vi "Begin.vi"(8 "error in":errorcluster) -> (0 "error out":errorcluster)   [LabVIEW 2017]
doc: "Called before other user functions, this VI is expected to open initial I/O refnums, load in file data, and do all program initialization. Notice that the <B>error out</B> terminal is simply used for data flow. Wiring it to other structures or subVIs ensures that this VI runs first."
uses:
  <vilib>/Rock Robotics/WPI/DriverStation/WPI_DriverStationRobotMode2.ctl
  <vilib>/Rock Robotics/WPI/Joystick/WPI_JoystickDeviceEnum.ctl
  Drive/Drive Notifier.ctl
  Drive/Drive Control Type.ctl
  Lift/Lift Notifier.ctl
  Lift/Lift Control Type.ctl
  Lift/Lift Enum States.ctl
  RPED/RPED Notifier.ctl
  RPED/RPED Control Type.ctl
  LEDs/LED Notifier.ctl
  LEDs/LED Control Type.ctl
  <vilib>/Rock Robotics/WPI/Solenoid/WPI_SolenoidChannel.ctl
  Intake Rotation/Intake Rotation Notifier.ctl
  Intake Rotation/Intake Rotation Control Type.ctl
  Intake Rotation/Arm Enum States.ctl
  Intake/Intake Notifier.ctl
  Intake/Intake Control Type.ctl
  <vilib>/Rock Robotics/SystemInterfaces/DIO/FPGA_DIOChannel.ctl
  <vilib>/Rock Robotics/WPI/ThirdParty/Phoenix-LabVIEW/Motor Controller/Controls/CTRE_Phoenix_MotorControl_FeedbackDevice.ctl
  <vilib>/Rock Robotics/SystemInterfaces/DIO/FPGA_DIOPWMChannel.ctl
  <vilib>/Rock Robotics/WPI/ThirdParty/Phoenix-LabVIEW/Motor Controller/Controls/CTRE_Phoenix_MotorControl_ControlMode.ctl
  Robot Global Data.vi
  <vilib>/Rock Robotics/WPI/Solenoid/WPI_SolenoidOpenDouble.vi
  <vilib>/Rock Robotics/WPI/ThirdParty/Phoenix-LabVIEW/Pigeon IMU/CTRE_PigeonIMU_Open_CAN.vi
  <vilib>/Rock Robotics/WPI/Switch/WPI_SwitchOpenLimit.vi
  <vilib>/Rock Robotics/WPI/MotorControl/WPI_MotorControlOpen VictorSP.vi
  Utility VIs/Refnum Names.vi
  Drive/Drive Globals.vi
  Intake/Intake Globals.vi
  Lift/Lift Globals.vi
  RPED/RPED Globals.vi
  Intake Rotation/Intake Rotation Globals.vi
  LEDs/LED Globals.vi
  <vilib>/Rock Robotics/WPI/Utilities/WPI_GetSetVariantRefNum.vi
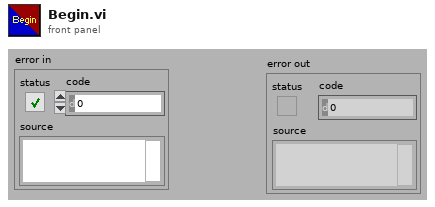
[diagram p1: front panel]
types:
  T1 = typedef "WPI_SolenoidChannel.ctl" = enum8{"Solenoid 0", "Solenoid 1", "Solenoid 2", "Solenoid 3", "Solenoid 4", "Solenoid 5", "Solenoid 6", "Solenoid 7", "Invalid"}
  T2 = enum16{"open", "replace", "create", "open or create", "replace or create", "replace or create with confirmation"}
  T3 = typedef "FPGA_DIOPWMChannel.ctl" = enum8{"PWM 0", "PWM 1", "PWM 2", "PWM 3", "PWM 4", "PWM 5", "PWM 6", "PWM 7", "PWM 8", "PWM 9", "PWM MXP 0", "PWM MXP 1", "PWM MXP 2", "PWM MXP 3", "PWM MXP 4", "PWM MXP 5", "PWM MXP 6", "PWM MXP 7", "PWM MXP 8", "PWM MXP 9", "Invalid"}
  T4 = typedef "FPGA_DIOChannel.ctl" = enum8{"DIO 0", "DIO 1", "DIO 2", "DIO 3", "DIO 4", "DIO 5", "DIO 6", "DIO 7", "DIO 8", "DIO 9", "DIO MXP 0", "DIO MXP 1", "DIO MXP 2", "DIO MXP 3", "DIO MXP 4", "DIO MXP 5", "DIO MXP 6", "DIO MXP 7", "DIO MXP 8", "DIO MXP 9", "DIO MXP 10", "DIO MXP 11", "DIO MXP 12", "DIO MXP 13", "DIO MXP 14", "DIO MXP 15", "SPI Port CS1", "SPI Port CS2", "SPI Port CS3", "SPI Port MISO", "SPI Port MOSI", "Invalid"}
  T5 = typedef "Intake Notifier.ctl" = cluster{"Intake Control Type":T6, "Step":i32, "In":bool, "Speed":dbl, "Out":bool, "Parameter 1":dbl, "Parameter 2":dbl, "Intake Notifier":refnum<notifier>, "Actuate Cube":bool, "Speed In":dbl, "Speed Out":dbl, "Load":bool, "Override":bool, "Exchange":bool, "Intake Open":bool}
  T6 = typedef "Intake Control Type.ctl" = enum16{"No Op", "In", "Out", "Test Mode", "Cube_In", "Cube_Out", "State_Change"}
  T7 = typedef "Intake Rotation Notifier.ctl" = cluster{"Step":i32, "Intake Rotation Control Type":T8, "Parameter 1":dbl, "Parameter 2":dbl, "Intake Rotation Notifier":refnum<notifier>, "Manual Up":bool, "Manual Down":bool, "Climb":bool, "Switch":bool, "Scale Low":bool, "Scale High":bool, "Stow":bool, "Load":bool, "Scale Mid":bool, "Exchange":bool, "Set Position":T9, "Portal":bool}
  T8 = typedef "Intake Rotation Control Type.ctl" = enum16{"No Op", "Manual Up", "Position", "Manual Down", "PositionAuto"}
  T9 = typedef "Arm Enum States.ctl" = enum16{"Current Position", "Climb", "Load", "Portal", "Switch", "Scale High", "Scale Mid", "Scale Low", "Exchange", "Stow"}
  T10 = typedef "LED Notifier.ctl" = cluster{"LED Control Type":T11, "Climbing":bool, "Auto Tracking":bool, "Ready for Cube Floor":bool, "Ready for Cube Portal":bool}
  T11 = typedef "LED Control Type.ctl" = enum16{"Off", "Waiting On Field", "Connected ", "Cube In Intake", "Climbing", "Auto Cube Capture", "Ready for Cube Floor", "Ready for Cube Portal"}
  T12 = typedef "RPED Notifier.ctl" = cluster{"RPED Control Type":T13, "Step":i32, "Left Forward":bool, "Right Forward":bool, "Parameter 1":dbl, "Parameter 2":dbl, "Parameter 3":dbl, "RPED Notifier":refnum<notifier>, "Left Back":bool, "Right Back":bool, "Right":bool, "Left":bool}
  T13 = typedef "RPED Control Type.ctl" = enum16{"No Op", "Left Manual", "Right Manual", "Time", "Left", "Right", "Left_Slow", "Right_Slow", "Left_Distance", "Right_Distance"}
  T14 = typedef "Lift Notifier.ctl" = cluster{"Lift Control Type":T15, "Step":i32, "Set Position":T16, "Climb":bool, "Switch":bool, "Scale Low":bool, "Scale Mid":bool, "Scale High":bool, "Stow":bool, "Load":bool, "Climb Actuation":bool, "Manual Up":bool, "Manual Down":bool, "Parameter 1":dbl, "Parameter 2":dbl, "Parameter 3":dbl, "Lift Notifier":refnum<notifier>, "Exchange":bool, "Brake":bool, "Portal":bool}
  T15 = typedef "Lift Control Type.ctl" = enum16{"No Op", "Position", "Climb Actuation", "Manual Up", "Manual Down", "PositionAuto", "Position_kP", "Position_Delay"}
  T16 = typedef "Lift Enum States.ctl" = enum16{"Climb", "Load", "Portal", "Switch", "Scale High", "Scale Mid", "Scale Low", "Exchange", "Stow", "Current Position"}
  T17 = typedef "Drive Notifier.ctl" = cluster{"Drive Control Type":T18, "Throttle":dbl, "Twist":dbl, "Step":i32, "High Gear":bool, "Parameter 1":dbl, "Parameter 2":dbl, "Parameter 3":dbl, "Drive Notifier":refnum<notifier>, "AutoTrack":bool}
  T18 = typedef "Drive Control Type.ctl" = enum16{"No_Op", "Basic Drive", "Time", "Heading", "Hybrid_Turn", "RC_Speed", "Switch_Slots", "AutoTrack_Cube", "Speed Test", "Turn_Cube", "To_Cube", "Wait", "Distance_Slow", "Distance", "D_H_Delay", "Distance_Delay", "Heading_Cap", "Heading_Tight", "Cube_Heading", "Distance_Ramp"}
  T19 = typedef "WPI_JoystickDeviceEnum.ctl" = enum16{"USB 0", "USB 1", "USB 2", "USB 3", "USB 4", "USB 5"}
  T20 = typedef "WPI_DriverStationRobotMode2.ctl" = enum16{"Autonomous Disabled", "Autonomous Enabled", "Teleop Disabled", "Teleop Enabled", "Disconnected", "Finish", "Test Disabled", "Test Enabled", "Emergency Stopped"}
  T21 = typedef "CTRE_Phoenix_MotorControl_FeedbackDevice.ctl" = i8
  T22 = typedef "CTRE_Phoenix_MotorControl_ControlMode.ctl" = u16
  T23 = typedef "WPI_MotorControlDeviceRef.ctl" = cluster{"DeviceStatus":errorcluster, "Type":T24, "PWM":cluster{"PWM Channel":T3, "DeadBand":T25}, "CAN":cluster{"Device Number":u8, "SetOutput VI Ref":variant, "GetOutput VI Ref":variant, "Enable VI Ref":variant, "Disable VI Ref":variant, "Data":variant}, "Invert":bool, "DIO PWM":cluster{"PWM \"Enable\" Channel":T3, "DIOChannel":T4, "PWM Rate":dbl}}
  T24 = typedef "WPI_MotorControlType.ctl" = enum16{"PWM", "CAN", "DIO PWM"}
  T25 = typedef "WPI_PWMDeadband.ctl" = cluster{"Name":string, "maxPositivePwm":i32, "minPositivePwm":i32, "centerPwm":i32, "maxNegativePwm":i32, "minNegativePwm":i32, "angularRange":u16}
  T26 = typedef "CTRE_PigeonIMU_DeviceRef.ctl" = cluster{"DeviceStatus":errorcluster, "Device Number":u8, "Type":T27, "Device ID":u32, "Handle":u64, "UsageFrame":u32, "Library Path":path}
  T27 = typedef "CTRE_PigeonIMU_ConnectionType.ctl" = u32
  T28 = typedef "CTRE_CANifier_DeviceRef.ctl" = cluster{"DeviceStatus":errorcluster, "Device Number":u8, "Handle":u64, "UsageFrame":u32, "Library Path":path}
  T29 = typedef "WPI_SwitchDevRef.ctl" = cluster{"DevStatus":errorcluster, "DIO Channel":T4, "CntIndex":T30, "Normally Closed":bool}
  T30 = typedef "FPGA_CounterCtrSystemIndex.ctl" = enum8{"Ctr 0", "Ctr 1", "Ctr 2", "Ctr 3", "Ctr 4", "Ctr 5", "Ctr 6", "Ctr 7", "Invalid"}
  T31 = typedef "WPI_SolenoidDevRef.ctl" = cluster{"DevStatus":errorcluster, "Pneumatics Control Module":u8, "Forward Solenoid Channel":T1, "Reverse Solenoid Channel":T1}
  T32 = typedef "WPI_DigitalInputDevRef.ctl" = cluster{"DevStatus":errorcluster, "DIO Channel":T4}
  T33 = typedef "WPI_CompressorDevRef.ctl" = cluster{"DevStatus":errorcluster, "Pneumatics Control Module":u8}
  T34 = typedef "WPI_JoystickDevRef.ctl" = cluster{"Device":T19}
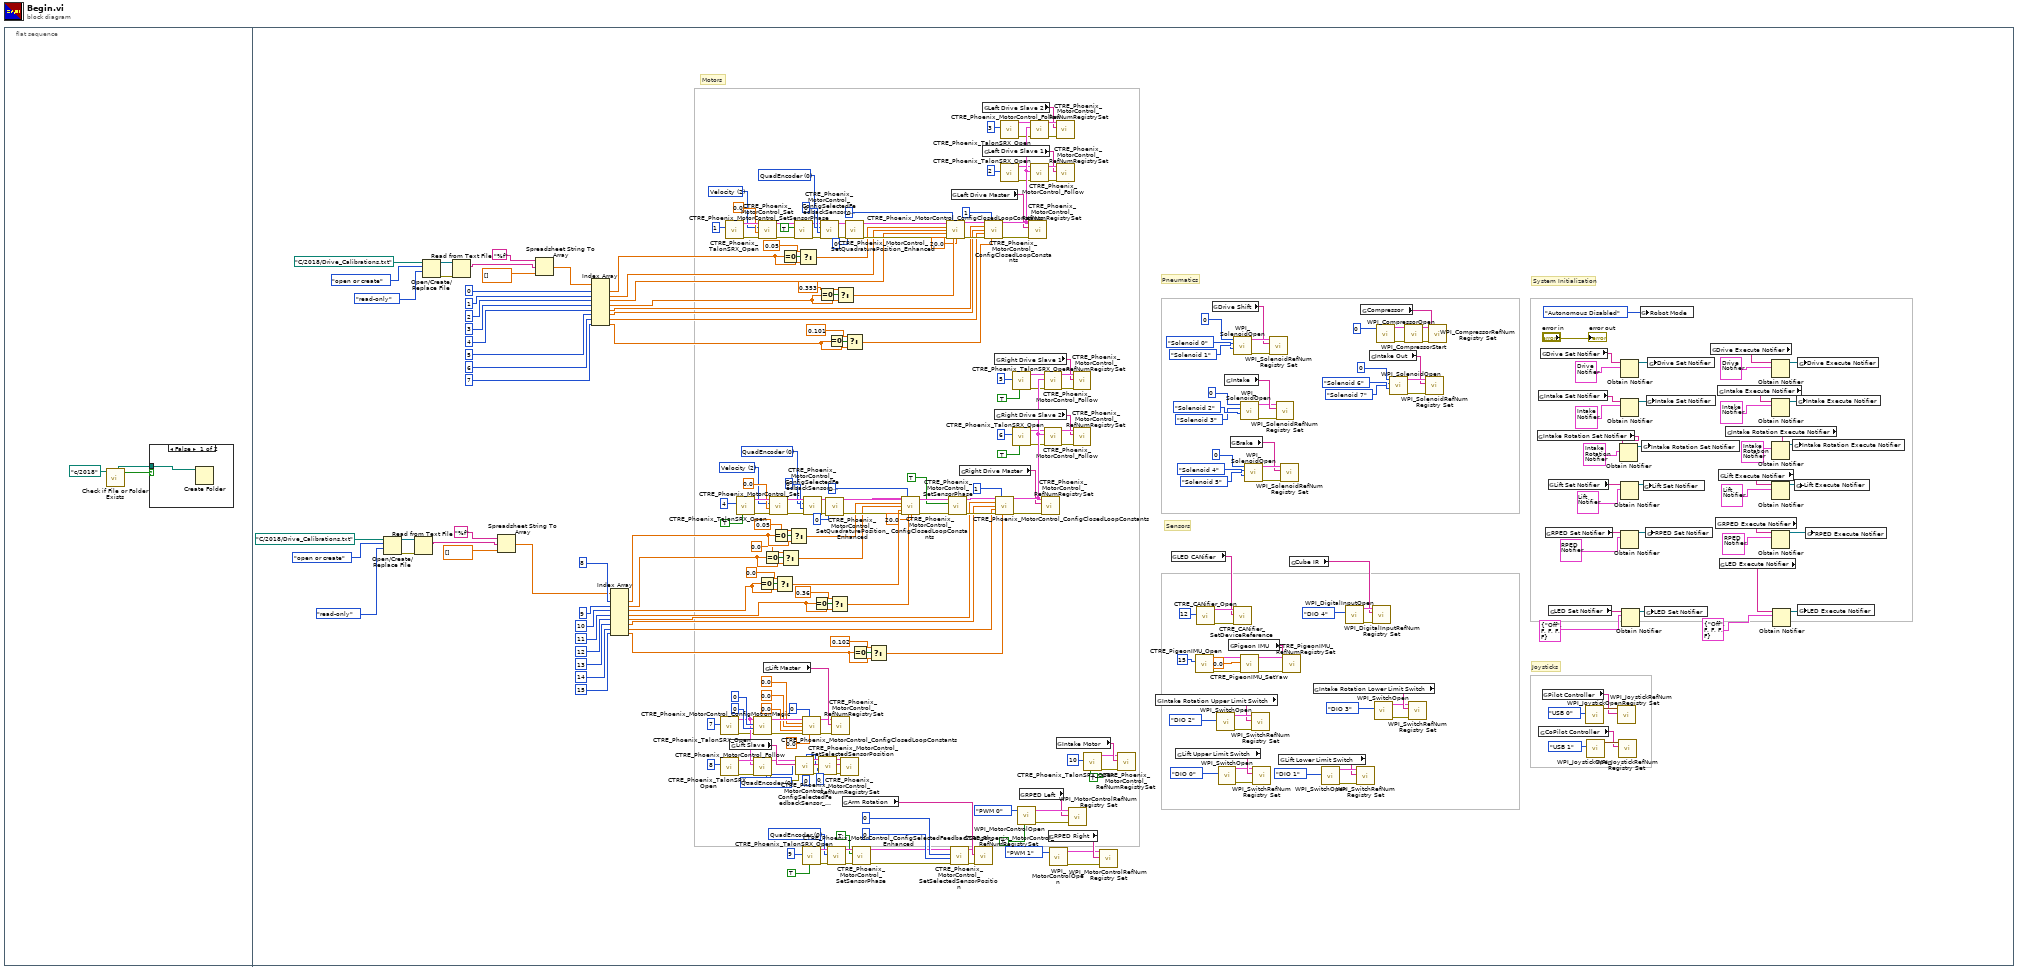
[diagram p0: block diagram]
diagram:
  n1 = flat-sequence {
    frame #0 {
      n2 = call <vilib>:"Check if File or Folder Exists.vi"("path"=path "c:/2018") -> ("file or folder exists?"=w3:bool, "dup path"=w1:path)  [unwired: 8 in, 1 out]
      n3 = case shown="False" w3 {
        tunnel: w1 -> [w4 _]
        frame False {
          n4 = Create Folder(path (use dialog)=w4) -> ()  [unwired: 2 in, 3 out]
        }
        frame True {
        }
      }
    }
    frame #1 {
      w111 = T21 0 items=["None"=-1, "QuadEncoder"=0, "Analog"=2, "Tachometer"=4, "Pulse Width Encoded Position"=8, "Sensor Sum (S0 + S1)"=9, "Sensor Difference (D0 - D1)"=10, "Remote Source 0"=11, "Remote Source 1"=12, "Software Emulated"=15] ("Feedback Device")
      w107 = T22 2 items=["PercentOutput"=0, "Position"=1, "Velocity"=2, "Current"=3, "Follower"=5, "MotionProfile"=6, "MotionMagic"=7, "MotionMagicArc"=8, "MotionProfileArc"=10, "Disabled"=15] ("Control Mode")
      w144 = T21 0 items=["None"=-1, "QuadEncoder"=0, "Analog"=2, "Tachometer"=4, "Pulse Width Encoded Position"=8, "Sensor Sum (S0 + S1)"=9, "Sensor Difference (D0 - D1)"=10, "Remote Source 0"=11, "Remote Source 1"=12, "Software Emulated"=15] ("Feedback Device")
      w140 = T22 2 items=["PercentOutput"=0, "Position"=1, "Velocity"=2, "Current"=3, "Follower"=5, "MotionProfile"=6, "MotionMagic"=7, "MotionMagicArc"=8, "MotionProfileArc"=10, "Disabled"=15] ("Control Mode")
      w204 = T21 0 items=["None"=-1, "QuadEncoder"=0, "Analog"=2, "Tachometer"=4, "Pulse Width Encoded Position"=8, "Sensor Sum (S0 + S1)"=9, "Sensor Difference (D0 - D1)"=10, "Remote Source 0"=11, "Remote Source 1"=12, "Software Emulated"=15] ("Feedback Device")
      w229 = T21 0 items=["None"=-1, "QuadEncoder"=0, "Analog"=2, "Tachometer"=4, "Pulse Width Encoded Position"=8, "Sensor Sum (S0 + S1)"=9, "Sensor Difference (D0 - D1)"=10, "Remote Source 0"=11, "Remote Source 1"=12, "Software Emulated"=15] ("Feedback Device")
      # "Joysticks"
      # "Sensors"
      # "System Initialization"
      # "Pneumatics"
      # "Motors"
      n5 = Open/Create/Replace File(file path (use dialog)=path "C:/2018/Drive_Calibrations.txt" ("file (use dialog)"), operation (0:open)=T2."open or create", access (0:read/write)=enum16{"read/write", "read-only", "write-only"}."read-only") -> (refnum out=w68:refnum<file>, error out=w67:errorcluster)  [unwired: 3 in, 1 out]
      n6 = Read from Text File(file (use dialog)=w68, error in=w67) -> (text=w61:string)  [unwired: 2 in, 3 out]
      n7 = Open/Create/Replace File(file path (use dialog)=path "C:/2018/Drive_Calibrations.txt" ("file (use dialog)"), operation (0:open)=T2."open or create", access (0:read/write)=enum16{"read/write", "read-only", "write-only"}."read-only") -> (refnum out=w59:refnum<file>, error out=w58:errorcluster)  [unwired: 3 in, 1 out]
      n8 = Read from Text File(file (use dialog)=w59, error in=w58) -> (text=w52:string)  [unwired: 2 in, 3 out]
      n9 = Spreadsheet String To Array(format string="%f", spreadsheet string=w61, array type (2D Dbl)=dbl[] []) -> (array=w60:dbl[])  [unwired: 1 in]
      n10 = Spreadsheet String To Array(format string="%f", spreadsheet string=w52, array type (2D Dbl)=dbl[] []) -> (array=w51:dbl[])  [unwired: 1 in]
      n11 = Index Array(array=w51, index #1=0 ("index"), index #2=1 ("index"), index #3=2 ("index"), index #4=3 ("index"), index #5=4 ("index"), index #6=5 ("index"), index #7=6 ("index"), index #8=7 ("index")) -> (element #1=w28:dbl, element #2=w84:dbl, element #3=w80:dbl, element #4=w23:dbl, element #5=w83:dbl, element #6=w82:dbl, element #7=w81:dbl, element #8=w19:dbl)
      n12 = Index Array(array=w60, index #1=8 ("index"), index #2=9 ("index"), index #3=10 ("index"), index #4=11 ("index"), index #5=12 ("index"), index #6=13 ("index"), index #7=14 ("index"), index #8=15 ("index")) -> (element #1=w49:dbl, element #2=w44:dbl, element #3=w41:dbl, element #4=w36:dbl, element #5=w71:dbl, element #6=w70:dbl, element #7=w69:dbl, element #8=w31:dbl)
      n13 = call <vilib>:"CTRE_Phoenix_TalonSRX_Open.vi"("Device Number"=u8 7) -> ("error out"=w263:errorcluster, "CAN Talon SRX Ref"=w264:T23)  [unwired: 9 in]
      n14 = call <vilib>:"CTRE_Phoenix_TalonSRX_Open.vi"("Device Number"=u8 8) -> ("error out"=w277:errorcluster, "CAN Talon SRX Ref"=w276:T23)  [unwired: 9 in]
      n15 = call <vilib>:"CTRE_Phoenix_TalonSRX_Open.vi"("Device Number"=u8 1) -> ("error out"=w117:errorcluster, "CAN Talon SRX Ref"=w118:T23)  [unwired: 9 in]
      n16 = global read "Refnum Names.vi" "Lift Slave"() -> (w279:string)
      n17 = call <vilib>:"CTRE_Phoenix_TalonSRX_Open.vi"("Invert"=TRUE, "Device Number"=u8 4) -> ("error out"=w155:errorcluster, "CAN Talon SRX Ref"=w156:T23)  [unwired: 8 in]
      n18 = call <vilib>:"CTRE_Phoenix_MotorControl_ConfigMotionMagic.vi"("error in (no error)"=w263, "Acceleration"=0, "Cruise Velocity"=0, "PhoenixMotorControlDevRef"=w264) -> ("error out"=w267:errorcluster, "PhoenixMotorControlDevRef"=w272:T23)  [unwired: 6 in]
      n19 = call <vilib>:"CTRE_Phoenix_MotorControl_Follow.vi"("error in (no error)"=w277, "Master Controller to Follow"=w264, "PhoenixMotorControlDevRef"=w276) -> ("error out"=w205:errorcluster, "PhoenixMotorControlDevRef"=w206:T23)  [unwired: 7 in]
      n20 = Equal To 0?(x=w41) -> (x = 0?=w42:bool)
      n21 = call <vilib>:"CTRE_Phoenix_MotorControl_Set.vi"("error in (no error)"=w117, "Output"=0.0, "Control Mode"=w107, "PhoenixMotorControlDevRef"=w118) -> ("error out"=w96:errorcluster, "PhoenixMotorControlDevRef"=w97:T23)  [unwired: 6 in]
      n22 = Equal To 0?(x=w44) -> (x = 0?=w45:bool)
      n23 = global read "Refnum Names.vi" "Lift Master"() -> (w280:string)
      n24 = call <vilib>:"CTRE_Phoenix_MotorControl_Set.vi"("error in (no error)"=w155, "Output"=0.0, "Control Mode"=w140, "PhoenixMotorControlDevRef"=w156) -> ("error out"=w151:errorcluster, "PhoenixMotorControlDevRef"=w152:T23)  [unwired: 6 in]
      n25 = Equal To 0?(x=w49) -> (x = 0?=w50:bool)
      n26 = Select(t=0.0, s=w42, f=w41) -> (s? t:f=w39:dbl)
      n27 = Equal To 0?(x=w28) -> (x = 0?=w30:bool)
      n28 = Select(t=0.0, s=w45, f=w44) -> (s? t:f=w43:dbl)
      n29 = Select(t=0.05, s=w50, f=w49) -> (s? t:f=w47:dbl)
      n30 = call <vilib>:"CTRE_Phoenix_MotorControl_SetSensorPhase.vi"("error in (no error)"=w96, "PhaseSensor"=TRUE, "PhoenixMotorControlDevRef"=w97) -> ("error out"=w95:errorcluster, "PhoenixMotorControlDevRef"=w94:T23)  [unwired: 7 in]
      n31 = call <vilib>:"CTRE_Phoenix_MotorControl_ConfigSelectedFeedbackSensor_Enhanced.vi"("error in (no error)"=w205, "Feedback Device"=w204, "PhoenixMotorControlDevRef"=w206) -> ("error out"=w188:errorcluster, "PhoenixMotorControlDevRef"=w189:T23)  [unwired: 7 in]
      n32 = Select(t=0.05, s=w30, f=w28) -> (s? t:f=w27:dbl)
      n33 = call <vilib>:"CTRE_Phoenix_TalonSRX_Open.vi"("Invert"=TRUE, "Device Number"=u8 9) -> ("error out"=w194:errorcluster, "CAN Talon SRX Ref"=w251:T23)  [unwired: 8 in]
      n34 = call <vilib>:"CTRE_Phoenix_MotorControl_ConfigClosedLoopConstants.vi"("PhoenixMotorControlDevRef"=w272, "slotIdx"=0, "P"=0.0, "I"=0.0, "D"=0.0, "error in (no error)"=w267, "F"=0.0) -> ("PhoenixMotorControlDevRef"=w265:T23, "error out"=w266:errorcluster)  [unwired: 7 in]
      n35 = call <vilib>:"CTRE_Phoenix_MotorControl_ConfigSelectedFeedbackSensor_Enhanced.vi"("error in (no error)"=w151, "pidLoopIdx"=0, "Feedback Device"=w144, "PhoenixMotorControlDevRef"=w152) -> ("error out"=w133:errorcluster, "PhoenixMotorControlDevRef"=w132:T23)  [unwired: 6 in]
      n36 = Equal To 0?(x=w36) -> (x = 0?=w38:bool)
      n37 = Equal To 0?(x=w23) -> (x = 0?=w26:bool)
      n38 = call <vilib>:"CTRE_Phoenix_MotorControl_SetSelectedSensorPosition.vi"("error in (no error)"=w188, "pidLoopIdx"=u32 0, "New Sensor Position"=0, "PhoenixMotorControlDevRef"=w189) -> ("error out"=w187:errorcluster, "PhoenixMotorControlDevRef"=w186:T23)  [unwired: 6 in]
      n39 = call <vilib>:"CTRE_Phoenix_MotorControl_ConfigSelectedFeedbackSensor_Enhanced.vi"("error in (no error)"=w95, "pidLoopIdx"=0, "Feedback Device"=w111, "PhoenixMotorControlDevRef"=w94) -> ("error out"=w101:errorcluster, "PhoenixMotorControlDevRef"=w102:T23)  [unwired: 6 in]
      n40 = call <vilib>:"CTRE_Phoenix_MotorControl_SetQuadraturePosition_Enhanced.vi"("error in (no error)"=w133, "New Position"=0, "PhoenixMotorControlDevRef"=w132) -> ("error out"=w130:errorcluster, "PhoenixMotorControlDevRef"=w131:T23)  [unwired: 7 in]
      n41 = call <vilib>:"CTRE_Phoenix_MotorControl_ConfigSelectedFeedbackSensor_Enhanced.vi"("error in (no error)"=w194, "Feedback Device"=w229, "PhoenixMotorControlDevRef"=w251) -> ("error out"=w209:errorcluster, "PhoenixMotorControlDevRef"=w208:T23)  [unwired: 7 in]
      n42 = Equal To 0?(x=w19) -> (x = 0?=w22:bool)
      n43 = Select(t=0.36, s=w38, f=w36) -> (s? t:f=w35:dbl)
      n44 = call <vilib>:"CTRE_Phoenix_MotorControl_RefNumRegistrySet.vi"("error in (no error)"=w266, "refnum name"=w280, "PhoenixMotorControlDevRef"=w265) -> ()  [unwired: 7 in, 2 out]
      n45 = Select(t=0.353, s=w26, f=w23) -> (s? t:f=w24:dbl)
      n46 = call <vilib>:"CTRE_Phoenix_MotorControl_RefNumRegistrySet.vi"("error in (no error)"=w187, "refnum name"=w279, "PhoenixMotorControlDevRef"=w186) -> ()  [unwired: 7 in, 2 out]
      n47 = global read "Refnum Names.vi" "Arm Rotation"() -> (w245:string)
      n48 = call <vilib>:"CTRE_Phoenix_MotorControl_SetQuadraturePosition_Enhanced.vi"("error in (no error)"=w101, "New Position"=0, "PhoenixMotorControlDevRef"=w102) -> ("error out"=w104:errorcluster, "PhoenixMotorControlDevRef"=w103:T23)  [unwired: 7 in]
      n49 = Select(t=0.101, s=w22, f=w19) -> (s? t:f=w21:dbl)
      n50 = Equal To 0?(x=w31) -> (x = 0?=w33:bool)
      n51 = call <vilib>:"CTRE_Phoenix_MotorControl_SetSensorPhase.vi"("error in (no error)"=w209, "PhaseSensor"=TRUE, "PhoenixMotorControlDevRef"=w208) -> ("error out"=w182:errorcluster, "PhoenixMotorControlDevRef"=w183:T23)  [unwired: 7 in]
      n52 = Select(t=0.102, s=w33, f=w31) -> (s? t:f=w32:dbl)
      n53 = call <vilib>:"CTRE_Phoenix_MotorControl_ConfigClosedLoopConstants.vi"("PhoenixMotorControlDevRef"=w131, "slotIdx"=0, "P"=w47, "I"=w43, "D"=w39, "error in (no error)"=w130, "F"=w35, "I Zone"=20.0) -> ("PhoenixMotorControlDevRef"=w149:T23, "error out"=w150:errorcluster)  [unwired: 6 in]
      n54 = call <vilib>:"CTRE_Phoenix_MotorControl_ConfigClosedLoopConstants.vi"("PhoenixMotorControlDevRef"=w103, "slotIdx"=0, "P"=w27, "I"=w84, "D"=w80, "error in (no error)"=w104, "F"=w24, "I Zone"=20.0) -> ("PhoenixMotorControlDevRef"=w99:T23, "error out"=w98:errorcluster)  [unwired: 6 in]
      n55 = call <vilib>:"CTRE_Phoenix_MotorControl_SetSensorPhase.vi"("error in (no error)"=w150, "PhaseSensor"=TRUE, "PhoenixMotorControlDevRef"=w149) -> ("error out"=w147:errorcluster, "PhoenixMotorControlDevRef"=w148:T23)  [unwired: 7 in]
      n56 = call <vilib>:"CTRE_Phoenix_MotorControl_SetSelectedSensorPosition.vi"("error in (no error)"=w182, "pidLoopIdx"=u32 0, "New Sensor Position"=0, "PhoenixMotorControlDevRef"=w183) -> ("error out"=w192:errorcluster, "PhoenixMotorControlDevRef"=w193:T23)  [unwired: 6 in]
      n57 = global read "Refnum Names.vi" "Left Drive Master"() -> (w115:string)
      n58 = global read "Refnum Names.vi" "Right Drive Master"() -> (w153:string)
      n59 = call <vilib>:"CTRE_Phoenix_MotorControl_RefNumRegistrySet.vi"("error in (no error)"=w192, "refnum name"=w245, "PhoenixMotorControlDevRef"=w193) -> ()  [unwired: 7 in, 2 out]
      n60 = global read "Refnum Names.vi" "Left Drive Slave 2"() -> (w114:string)
      n61 = global read "Refnum Names.vi" "Left Drive Slave 1"() -> (w119:string)
      n62 = call <vilib>:"CTRE_Phoenix_MotorControl_ConfigClosedLoopConstants.vi"("PhoenixMotorControlDevRef"=w99, "slotIdx"=1, "P"=w83, "I"=w82, "D"=w81, "error in (no error)"=w98, "F"=w21) -> ("PhoenixMotorControlDevRef"=w128:T23, "error out"=w116:errorcluster)  [unwired: 7 in]
      n63 = global read "Refnum Names.vi" "Right Drive Slave 1"() -> (w158:string)
      n64 = global read "Refnum Names.vi" "Right Drive Slave 2"() -> (w157:string)
      n65 = call <vilib>:"CTRE_Phoenix_MotorControl_ConfigClosedLoopConstants.vi"("PhoenixMotorControlDevRef"=w148, "slotIdx"=1, "P"=w71, "I"=w70, "D"=w69, "error in (no error)"=w147, "F"=w32) -> ("PhoenixMotorControlDevRef"=w165:T23, "error out"=w154:errorcluster)  [unwired: 7 in]
      n66 = call <vilib>:"CTRE_Phoenix_TalonSRX_Open.vi"("Device Number"=u8 3) -> ("error out"=w120:errorcluster, "CAN Talon SRX Ref"=w121:T23)  [unwired: 9 in]
      n67 = call <vilib>:"CTRE_Phoenix_TalonSRX_Open.vi"("Device Number"=u8 2) -> ("error out"=w125:errorcluster, "CAN Talon SRX Ref"=w124:T23)  [unwired: 9 in]
      n68 = call <vilib>:"CTRE_Phoenix_TalonSRX_Open.vi"("Invert"=TRUE, "Device Number"=u8 5) -> ("error out"=w164:errorcluster, "CAN Talon SRX Ref"=w163:T23)  [unwired: 8 in]
      n69 = call <vilib>:"CTRE_Phoenix_TalonSRX_Open.vi"("Invert"=TRUE ("Enable Current Limit?"), "Device Number"=u8 6) -> ("error out"=w160:errorcluster, "CAN Talon SRX Ref"=w159:T23)  [unwired: 8 in]
      n70 = call-poly <vilib>:"WPI_MotorControlOpen.vi"("Invert"=TRUE, "PWM Channel"=FPGA_DIOPWMChannel."PWM 0") -> ("error out"=w181:errorcluster, "MotorControlDeviceRef"=w180:T23)  [unwired: 8 in]
      n71 = global read "Refnum Names.vi" "RPED Left"() -> (w178:string)
      n72 = call <vilib>:"CTRE_Phoenix_MotorControl_RefNumRegistrySet.vi"("error in (no error)"=w116, "refnum name"=w115, "PhoenixMotorControlDevRef"=w128) -> ()  [unwired: 7 in, 2 out]
      n73 = call <vilib>:"CTRE_Phoenix_MotorControl_Follow.vi"("error in (no error)"=w120, "Master Controller to Follow"=w128, "PhoenixMotorControlDevRef"=w121) -> ("error out"=w123:errorcluster, "PhoenixMotorControlDevRef"=w122:T23)  [unwired: 7 in]
      n74 = call <vilib>:"CTRE_Phoenix_MotorControl_Follow.vi"("error in (no error)"=w125, "Master Controller to Follow"=w128, "PhoenixMotorControlDevRef"=w124) -> ("error out"=w127:errorcluster, "PhoenixMotorControlDevRef"=w126:T23)  [unwired: 7 in]
      n75 = call <vilib>:"CTRE_Phoenix_MotorControl_RefNumRegistrySet.vi"("error in (no error)"=w154, "refnum name"=w153, "PhoenixMotorControlDevRef"=w165) -> ()  [unwired: 7 in, 2 out]
      n76 = call <vilib>:"CTRE_Phoenix_MotorControl_Follow.vi"("error in (no error)"=w164, "Master Controller to Follow"=w165, "PhoenixMotorControlDevRef"=w163) -> ("error out"=w167:errorcluster, "PhoenixMotorControlDevRef"=w166:T23)  [unwired: 7 in]
      n77 = call <vilib>:"CTRE_Phoenix_MotorControl_Follow.vi"("error in (no error)"=w160, "Master Controller to Follow"=w165, "PhoenixMotorControlDevRef"=w159) -> ("error out"=w161:errorcluster, "PhoenixMotorControlDevRef"=w162:T23)  [unwired: 7 in]
      n78 = global read "Refnum Names.vi" "RPED Right"() -> (w177:string)
      n79 = call-poly <vilib>:"WPI_MotorControlOpen.vi"("PWM Channel"=FPGA_DIOPWMChannel."PWM 1") -> ("error out"=w174:errorcluster, "MotorControlDeviceRef"=w175:T23)  [unwired: 9 in]
      n80 = call <vilib>:"CTRE_Phoenix_MotorControl_RefNumRegistrySet.vi"("error in (no error)"=w123, "refnum name"=w114, "PhoenixMotorControlDevRef"=w122) -> ()  [unwired: 7 in, 2 out]
      n81 = call <vilib>:"CTRE_Phoenix_MotorControl_RefNumRegistrySet.vi"("error in (no error)"=w127, "refnum name"=w119, "PhoenixMotorControlDevRef"=w126) -> ()  [unwired: 7 in, 2 out]
      n82 = global read "Refnum Names.vi" "Intake Motor"() -> (w231:string)
      n83 = call <vilib>:"WPI_MotorControlRefNum Registry Set.vi"("error in (no error)"=w181, "refnum name"=w178, "MotorControlDevRef"=w180) -> ()  [unwired: 7 in, 2 out]
      n84 = call <vilib>:"CTRE_Phoenix_MotorControl_RefNumRegistrySet.vi"("error in (no error)"=w167, "refnum name"=w158, "PhoenixMotorControlDevRef"=w166) -> ()  [unwired: 7 in, 2 out]
      n85 = call <vilib>:"CTRE_Phoenix_MotorControl_RefNumRegistrySet.vi"("error in (no error)"=w161, "refnum name"=w157, "PhoenixMotorControlDevRef"=w162) -> ()  [unwired: 7 in, 2 out]
      n86 = call <vilib>:"CTRE_Phoenix_TalonSRX_Open.vi"("Invert"=TRUE, "Device Number"=u8 10) -> ("error out"=w211:errorcluster, "CAN Talon SRX Ref"=w212:T23)  [unwired: 8 in]
      n87 = call <vilib>:"WPI_MotorControlRefNum Registry Set.vi"("error in (no error)"=w174, "refnum name"=w177, "MotorControlDevRef"=w175) -> ()  [unwired: 7 in, 2 out]
      n88 = call <vilib>:"CTRE_Phoenix_MotorControl_RefNumRegistrySet.vi"("error in (no error)"=w211, "refnum name"=w231, "PhoenixMotorControlDevRef"=w212) -> ()  [unwired: 7 in, 2 out]
      n89 = global read "Refnum Names.vi" "Intake Rotation Upper Limit Switch"() -> (w221:string)
      n90 = global read "Refnum Names.vi" "LED CANifier"() -> (w246:string)
      n91 = global read "Refnum Names.vi" "Lift Upper Limit Switch"() -> (w220:string)
      n92 = call-poly <vilib>:"CTRE_PigeonIMU_Open.vi"("Device Number"=u8 15) -> ("error out"=w171:errorcluster, "PigeonIMUDevRef"=w172:T26)  [unwired: 9 in]
      n93 = call <vilib>:"CTRE_CANifier_Open.vi"("Device Number"=u8 12) -> ("error out"=w248:errorcluster, "CANifierDevRef"=w249:T28)  [unwired: 9 in]
      n94 = global read "Refnum Names.vi" "Drive Shift"() -> (w244:string)
      n95 = call-poly <vilib>:"WPI_SwitchOpen.vi"("DIO Channel"=FPGA_DIOChannel."DIO 2") -> ("error out"=w222:errorcluster, "SwitchDevRef"=w223:T29)  [unwired: 9 in]
      n96 = call-poly <vilib>:"WPI_SwitchOpen.vi"("DIO Channel"=FPGA_DIOChannel."DIO 0") -> ("error out"=w219:errorcluster, "SwitchDevRef"=w218:T29)  [unwired: 9 in]
      n97 = global read "Refnum Names.vi" "Intake"() -> (w243:string)
      n98 = global read "Refnum Names.vi" "Pigeon IMU"() -> (w227:string)
      n99 = global read "Refnum Names.vi" "Brake"() -> (w232:string)
      n100 = call <vilib>:"CTRE_CANifier_SetDeviceReference.vi"("error in (no error)"=w248, "refnum name"=w246, "CANifierDevRef"=w249) -> ()  [unwired: 7 in, 2 out]
      n101 = call-poly <vilib>:"WPI_SolenoidOpen.vi"("Reverse Solenoid Channel"=WPI_SolenoidChannel."Solenoid 0", "Forward Solenoid Channel"=WPI_SolenoidChannel."Solenoid 1" ("Solenoid Channel"), "Pneumatics Control Module (0)"=u8 0) -> ("error out"=w256:errorcluster, "SolenoidDevRef"=w255:T31)  [unwired: 7 in]
      n102 = call-poly <vilib>:"WPI_SolenoidOpen.vi"("Reverse Solenoid Channel"=WPI_SolenoidChannel."Solenoid 2", "Forward Solenoid Channel"=WPI_SolenoidChannel."Solenoid 3" ("Solenoid Channel"), "Pneumatics Control Module (0)"=u8 0) -> ("error out"=w238:errorcluster, "SolenoidDevRef"=w239:T31)  [unwired: 7 in]
      n103 = call <vilib>:"CTRE_PigeonIMU_SetYaw.vi"("error in (no error)"=w171, "Value"=0.0, "PigeonIMUDevRef"=w172) -> ("error out"=w170:errorcluster, "PigeonIMUDevRef"=w169:T26)  [unwired: 7 in]
      n104 = call-poly <vilib>:"WPI_SolenoidOpen.vi"("Reverse Solenoid Channel"=WPI_SolenoidChannel."Solenoid 4", "Forward Solenoid Channel"=WPI_SolenoidChannel."Solenoid 5" ("Solenoid Channel"), "Pneumatics Control Module (0)"=u8 0) -> ("error out"=w237:errorcluster, "SolenoidDevRef"=w236:T31)  [unwired: 7 in]
      n105 = call <vilib>:"WPI_SwitchRefNum Registry Set.vi"("error in (no error)"=w222, "refnum name"=w221, "SwitchDevRef"=w223) -> ()  [unwired: 7 in, 2 out]
      n106 = call <vilib>:"WPI_SwitchRefNum Registry Set.vi"("error in (no error)"=w219, "refnum name"=w220, "SwitchDevRef"=w218) -> ()  [unwired: 7 in, 2 out]
      n107 = call <vilib>:"WPI_SolenoidRefNum Registry Set.vi"("error in (no error)"=w256, "refnum name"=w244, "SolenoidDevRef"=w255) -> ()  [unwired: 7 in, 2 out]
      n108 = call <vilib>:"WPI_SolenoidRefNum Registry Set.vi"("error in (no error)"=w238, "refnum name"=w243, "SolenoidDevRef"=w239) -> ()  [unwired: 7 in, 2 out]
      n109 = global read "Refnum Names.vi" "Lift Lower Limit Switch"() -> (w213:string)
      n110 = call <vilib>:"WPI_SolenoidRefNum Registry Set.vi"("error in (no error)"=w237, "refnum name"=w232, "SolenoidDevRef"=w236) -> ()  [unwired: 7 in, 2 out]
      n111 = call <vilib>:"CTRE_PigeonIMU_RefNumRegistrySet.vi"("error in (no error)"=w170, "refnum name"=w227, "PigeonIMUDevRef"=w169) -> ()  [unwired: 7 in, 2 out]
      n112 = global read "Refnum Names.vi" "Cube IR"() -> (w197:string)
      n113 = global read "Refnum Names.vi" "Intake Rotation Lower Limit Switch"() -> (w203:string)
      n114 = call-poly <vilib>:"WPI_SwitchOpen.vi"("DIO Channel"=FPGA_DIOChannel."DIO 1") -> ("error out"=w214:errorcluster, "SwitchDevRef"=w215:T29)  [unwired: 9 in]
      n115 = call <vilib>:"WPI_DigitalInputOpen.vi"("DIO Channel"=FPGA_DIOChannel."DIO 4") -> ("error out"=w199:errorcluster, "DigitalInputDevRef"=w198:T32)  [unwired: 9 in]
      n116 = call <vilib>:"WPI_SwitchRefNum Registry Set.vi"("error in (no error)"=w214, "refnum name"=w213, "SwitchDevRef"=w215) -> ()  [unwired: 7 in, 2 out]
      n117 = global read "Refnum Names.vi" "Compressor"() -> (w16:string)
      n118 = global read "Refnum Names.vi" "Intake Out"() -> (w5:string)
      n119 = call <vilib>:"WPI_DigitalInputRefNum Registry Set.vi"("error in (no error)"=w199, "refnum name"=w197, "DigitalInputDevRef"=w198) -> ()  [unwired: 7 in, 2 out]
      n120 = call-poly <vilib>:"WPI_SwitchOpen.vi"("DIO Channel"=FPGA_DIOChannel."DIO 3") -> ("error out"=w202:errorcluster, "SwitchDevRef"=w201:T29)  [unwired: 9 in]
      n121 = call <vilib>:"WPI_CompressorOpen.vi"("Pneumatics Control Module (0)"=u8 0) -> ("CompressorDevRef"=w14:T33, "error out"=w13:errorcluster)  [unwired: 13 in]
      n122 = call-poly <vilib>:"WPI_SolenoidOpen.vi"("Reverse Solenoid Channel"=WPI_SolenoidChannel."Solenoid 6", "Forward Solenoid Channel"=WPI_SolenoidChannel."Solenoid 7" ("Solenoid Channel"), "Pneumatics Control Module (0)"=u8 0) -> ("error out"=w7:errorcluster, "SolenoidDevRef"=w8:T31)  [unwired: 7 in]
      n123 = call <vilib>:"WPI_CompressorStart.vi"("error in (no error)"=w13, "CompressorDevRef"=w14) -> ("error out"=w12:errorcluster, "CompressorDevRef"=w11:T33)  [unwired: 8 in]
      n124 = call <vilib>:"WPI_SwitchRefNum Registry Set.vi"("error in (no error)"=w202, "refnum name"=w203, "SwitchDevRef"=w201) -> ()  [unwired: 7 in, 2 out]
      n125 = call <vilib>:"WPI_SolenoidRefNum Registry Set.vi"("error in (no error)"=w7, "refnum name"=w5, "SolenoidDevRef"=w8) -> ()  [unwired: 7 in, 2 out]
      n126 = call <vilib>:"WPI_CompressorRefNum Registry Set.vi"("error in (no error)"=w12, "refnum name"=w16, "CompressorDevRef"=w11) -> ()  [unwired: 7 in, 2 out]
      n127 = global read "Refnum Names.vi" "Intake Rotation Set Notifier"() -> (w284:string)
      n128 = global read "Refnum Names.vi" "Intake Set Notifier"() -> (w307:string)
      n129 = global read "Refnum Names.vi" "CoPilot Controller"() -> (w310:string)
      n130 = global read "Refnum Names.vi" "Drive Set Notifier"() -> (w309:string)
      n131 = global read "Refnum Names.vi" "Pilot Controller"() -> (w311:string)
      n132 = global read "Refnum Names.vi" "RPED Set Notifier"() -> (w290:string)
      n133 = global read "Refnum Names.vi" "Lift Set Notifier"() -> (w305:string)
      n134 = global read "Refnum Names.vi" "LED Set Notifier"() -> (w262:string)
      n135 = call <vilib>:"WPI_JoystickOpen.vi"("JoystickDevice"=WPI_JoystickDeviceEnum."USB 0") -> ("JoystickDevRef"=w315:T34)  [unwired: 10 in]
      n136 = call <vilib>:"WPI_JoystickOpen.vi"("JoystickDevice"=WPI_JoystickDeviceEnum."USB 1") -> ("JoystickDevRef"=w312:T34)  [unwired: 10 in]
      n137 = call <vilib>:"WPI_JoystickRefNum Registry Set.vi"("refnum name"=w311, "JoystickDevRef"=w315) -> ()  [unwired: 8 in, 2 out]
      n138 = call <vilib>:"WPI_JoystickRefNum Registry Set.vi"("refnum name"=w310, "JoystickDevRef"=w312) -> ()  [unwired: 8 in, 2 out]
      n139 = Obtain Notifier(name (unnamed)=w284, notification data type=T7 {"Step"=0, "Intake Rotation Control Type"=enum."No Op", "Parameter 1"=0.0, "Parameter 2"=0.0, "Intake Rotation Notifier"=refnum, "Manual Up"=FALSE, "Manual Down"=FALSE, "Climb"=FALSE, "Switch"=FALSE, "Scale Low"=FALSE, "Scale High"=FALSE, "Stow"=FALSE, "Load"=FALSE, "Scale Mid"=FALSE, "Exchange"=FALSE, "Set Position"=enum."Climb", "Portal"=FALSE} ("Intake Rotation Notifier")) -> (notifier out=w225:refnum<notifier>)  [unwired: 2 in, 2 out]
      n140 = Obtain Notifier(name (unnamed)=w309, notification data type=T17 {"Drive Control Type"=enum."No_Op", "Throttle"=0.0, "Twist"=0.0, "Step"=0, "High Gear"=FALSE, "Parameter 1"=0.0, "Parameter 2"=0.0, "Parameter 3"=0.0, "Drive Notifier"=refnum, "AutoTrack"=FALSE} ("Drive Notifier")) -> (notifier out=w300:refnum<notifier>)  [unwired: 2 in, 2 out]
      n141 = Obtain Notifier(name (unnamed)=w307, notification data type=T5 {"Intake Control Type"=enum."No Op", "Step"=0, "In"=FALSE, "Speed"=0.0, "Out"=FALSE, "Parameter 1"=0.0, "Parameter 2"=0.0, "Intake Notifier"=refnum, "Actuate Cube"=FALSE, "Speed In"=0.0, "Speed Out"=0.0, "Load"=FALSE, "Override"=FALSE, "Exchange"=FALSE, "Intake Open"=FALSE} ("Intake Notifier")) -> (notifier out=w295:refnum<notifier>)  [unwired: 2 in, 2 out]
      n142 = Obtain Notifier(name (unnamed)=w305, notification data type=T14 {"Lift Control Type"=enum."No Op", "Step"=0, "Set Position"=enum."Load", "Climb"=FALSE, "Switch"=FALSE, "Scale Low"=FALSE, "Scale Mid"=FALSE, "Scale High"=FALSE, "Stow"=FALSE, "Load"=FALSE, "Climb Actuation"=FALSE, "Manual Up"=FALSE, "Manual Down"=FALSE, "Parameter 1"=0.0, "Parameter 2"=0.0, "Parameter 3"=0.0, "Lift Notifier"=refnum, "Exchange"=FALSE, "Brake"=FALSE, "Portal"=FALSE} ("Lift Notifier")) -> (notifier out=w292:refnum<notifier>)  [unwired: 2 in, 2 out]
      n143 = Obtain Notifier(name (unnamed)=w290, notification data type=T12 {"RPED Control Type"=enum."No Op", "Step"=0, "Left Forward"=FALSE, "Right Forward"=FALSE, "Parameter 1"=0.0, "Parameter 2"=0.0, "Parameter 3"=0.0, "RPED Notifier"=refnum, "Left Back"=FALSE, "Right Back"=FALSE, "Right"=FALSE, "Left"=FALSE} ("RPED Notifier")) -> (notifier out=w287:refnum<notifier>)  [unwired: 2 in, 2 out]
      n144 = Obtain Notifier(name (unnamed)=w262, notification data type=T10 {"LED Control Type"=enum."Off", "Climbing"=FALSE, "Auto Tracking"=FALSE, "Ready for Cube Floor"=FALSE, "Ready for Cube Portal"=FALSE} ("LED Notifier")) -> (notifier out=w258:refnum<notifier>)  [unwired: 2 in, 2 out]
      n145 = global write "Robot Global Data.vi" "Robot Mode"(WPI_DriverStationRobotMode2."Autonomous Disabled" ("Robot Mode")) -> ()
      n146 = global write "Intake Rotation Globals.vi" "Intake Rotation Set Notifier"(w225) -> ()
      n147 = global write "Lift Globals.vi" "Lift Set Notifier"(w292) -> ()
      n148 = global write "LED Globals.vi" "LED Set Notifier"(w258) -> ()
      n149 = global write "RPED Globals.vi" "RPED Set Notifier"(w287) -> ()
      n150 = global write "Intake Globals.vi" "Intake Set Notifier"(w295) -> ()
      n151 = global write "Drive Globals.vi" "Drive Set Notifier"(w300) -> ()
      n152 = global read "Refnum Names.vi" "Drive Execute Notifier"() -> (w308:string)
      n153 = global read "Refnum Names.vi" "RPED Execute Notifier"() -> (w291:string)
      n154 = global read "Refnum Names.vi" "Intake Execute Notifier"() -> (w306:string)
      n155 = global read "Refnum Names.vi" "Lift Execute Notifier"() -> (w304:string)
      n156 = global read "Refnum Names.vi" "LED Execute Notifier"() -> (w261:string)
      n157 = global read "Refnum Names.vi" "Intake Rotation Execute Notifier"() -> (w285:string)
      n158 = Obtain Notifier(name (unnamed)=w308, notification data type=T17 {"Drive Control Type"=enum."No_Op", "Throttle"=0.0, "Twist"=0.0, "Step"=0, "High Gear"=FALSE, "Parameter 1"=0.0, "Parameter 2"=0.0, "Parameter 3"=0.0, "Drive Notifier"=refnum, "AutoTrack"=FALSE} ("Drive Notifier")) -> (notifier out=w301:refnum<notifier>)  [unwired: 2 in, 2 out]
      n159 = Obtain Notifier(name (unnamed)=w306, notification data type=T5 {"Intake Control Type"=enum."No Op", "Step"=0, "In"=FALSE, "Speed"=0.0, "Out"=FALSE, "Parameter 1"=0.0, "Parameter 2"=0.0, "Intake Notifier"=refnum, "Actuate Cube"=FALSE, "Speed In"=0.0, "Speed Out"=0.0, "Load"=FALSE, "Override"=FALSE, "Exchange"=FALSE, "Intake Open"=FALSE} ("Intake Notifier")) -> (notifier out=w294:refnum<notifier>)  [unwired: 2 in, 2 out]
      n160 = Obtain Notifier(name (unnamed)=w304, notification data type=T14 {"Lift Control Type"=enum."No Op", "Step"=0, "Set Position"=enum."Load", "Climb"=FALSE, "Switch"=FALSE, "Scale Low"=FALSE, "Scale Mid"=FALSE, "Scale High"=FALSE, "Stow"=FALSE, "Load"=FALSE, "Climb Actuation"=FALSE, "Manual Up"=FALSE, "Manual Down"=FALSE, "Parameter 1"=0.0, "Parameter 2"=0.0, "Parameter 3"=0.0, "Lift Notifier"=refnum, "Exchange"=FALSE, "Brake"=FALSE, "Portal"=FALSE} ("Lift Notifier")) -> (notifier out=w293:refnum<notifier>)  [unwired: 2 in, 2 out]
      n161 = Obtain Notifier(name (unnamed)=w291, notification data type=T12 {"RPED Control Type"=enum."No Op", "Step"=0, "Left Forward"=FALSE, "Right Forward"=FALSE, "Parameter 1"=0.0, "Parameter 2"=0.0, "Parameter 3"=0.0, "RPED Notifier"=refnum, "Left Back"=FALSE, "Right Back"=FALSE, "Right"=FALSE, "Left"=FALSE} ("RPED Notifier")) -> (notifier out=w286:refnum<notifier>)  [unwired: 2 in, 2 out]
      n162 = Obtain Notifier(name (unnamed)=w285, notification data type=T7 {"Step"=0, "Intake Rotation Control Type"=enum."No Op", "Parameter 1"=0.0, "Parameter 2"=0.0, "Intake Rotation Notifier"=refnum, "Manual Up"=FALSE, "Manual Down"=FALSE, "Climb"=FALSE, "Switch"=FALSE, "Scale Low"=FALSE, "Scale High"=FALSE, "Stow"=FALSE, "Load"=FALSE, "Scale Mid"=FALSE, "Exchange"=FALSE, "Set Position"=enum."Climb", "Portal"=FALSE} ("Intake Rotation Notifier")) -> (notifier out=w282:refnum<notifier>)  [unwired: 2 in, 2 out]
      n163 = Obtain Notifier(name (unnamed)=w261, notification data type=T10 {"LED Control Type"=enum."Off", "Climbing"=FALSE, "Auto Tracking"=FALSE, "Ready for Cube Floor"=FALSE, "Ready for Cube Portal"=FALSE} ("LED Notifier")) -> (notifier out=w257:refnum<notifier>)  [unwired: 2 in, 2 out]
      n164 = global write "Intake Rotation Globals.vi" "Intake Rotation Execute Notifier"(w282) -> ()
      n165 = global write "Lift Globals.vi" "Lift Execute Notifier"(w293) -> ()
      n166 = global write "Intake Globals.vi" "Intake Execute Notifier"(w294) -> ()
      n167 = global write "Drive Globals.vi" "Drive Execute Notifier"(w301) -> ()
      n168 = global write "LED Globals.vi" "LED Execute Notifier"(w257) -> ()
      n169 = global write "RPED Globals.vi" "RPED Execute Notifier"(w286) -> ()
      "error out" <- "error in"
    }
  }
